vi "ProSCI ConfigGlobal.vi"() -> ()   [LabVIEW 2012]
panel:
  out "gCfgMicronPerMicronThickness":dbl
  out "gCfgPixelSize":dbl[][](array[numeric])
  out "gCfgMicronPerStep":dbl
  # "Robot Configuration Settings"
  # "Camera Configuration Settings"
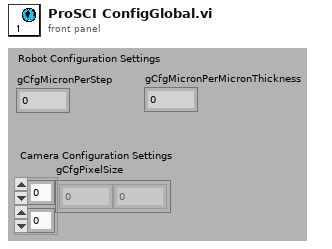
[diagram p1: front panel]
diagram:
